vi "GUI.SelectPageInMainTab.vi"(8 "error in (no error)":errorcluster, 10 "pageNumber":i32, 11 "referenceToControls in":refnum<vi>[](array[refnum])) -> (0 "error out":errorcluster, 3 "referenceToControls out":refnum<vi>[](array[refnum]))   [LabVIEW 2019]
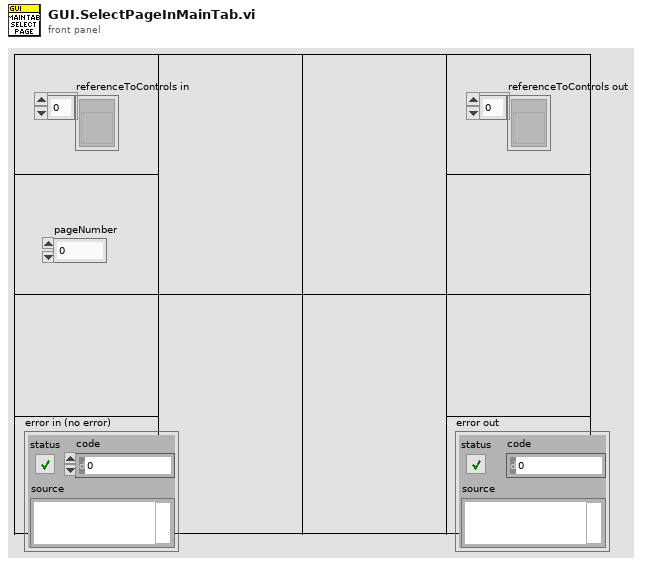
[diagram p1: front panel]
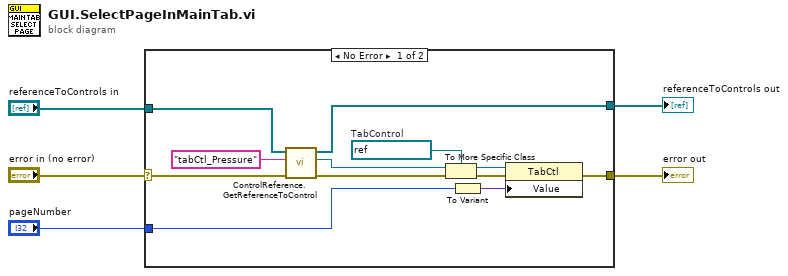
[diagram p0: block diagram]
diagram:
  n1 = case shown="No Error" "error in (no error)" {
    selector: "error in (no error)" -> [w11 w19]
    tunnel: [w16 w19] -> w4
    tunnel: "referenceToControls in" -> [w7 w18]
    tunnel: [w8 w18] -> w2
    tunnel: "pageNumber" -> [w6 _]
    frame No Error {
      w15 = refnum<vi> refnum  # TabControl
      n2 = call "ControlReference.GetReferenceToControl.vi"("error in (no error)"=w11, "controlLabelText"="tabCtl_Pressure", "referenceToControls in"=w7) -> ("error out"=w10:errorcluster, "referenceToControl"=w9:refnum<vi>, "referenceToControls out"=w8:refnum<vi>[])  [unwired: 6 in]
      n3 = To More Specific Class(target class=w15, reference=w9, error in=w10) -> (specific class reference=w14:refnum<vi>, error out=w17:errorcluster)
      n4 = To Variant(anything=w6) -> (Variant=w13:variant)
      n5 = property class="TabCtl"(reference=w14, error in=w17, "Value"=w13) -> (error out=w16:errorcluster)  [unwired: 1 out]
    }
    frame Error {
    }
  }
  "error out" <- w4
  "referenceToControls out" <- w2
